vi "Handle.vi"(7 "Queue Actor in":refnum<class "Queue Actor.lvclass">, 11 "Teardown State in":refnum<class "Teardown State.lvclass">) -> (2 "Destroy?":bool, 5 "Queue Actor out":refnum<class "Queue Actor.lvclass">)   [LabVIEW 2021, in "jettl.lvlib" / "Teardown State.lvclass"]
uses:
  Teardown State.lvclass
  Queue Actor/Queue Actor.lvclass
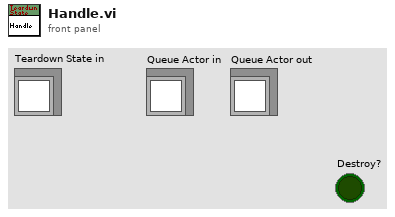
[diagram p1: front panel]
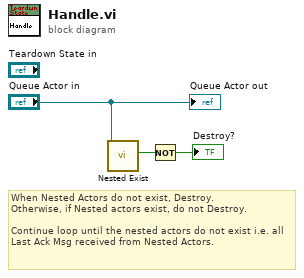
[diagram p0: block diagram]
diagram:
  # "When Nested Actors do not exist, Destroy.\nOtherwise, if Nested actors exist, do not Destroy.\n\nContinue loop until the nested actors do not exist i.e. all Last Ack Msg received from Nested Actors."
  n1 = call-dynamic "Nested Exist.vi"("Queue Actor in"="Queue Actor in") -> ("Nested Exist?"=w3:bool)  [unwired: 10 in]
  n2 = Not(x=w3) -> (.not. x?=→"Destroy?":bool)
  "Queue Actor out" <- "Queue Actor in"
